vi "Initialize Page Number.vi"(8 "error in (no error)":errorcluster, 11 "Test Node Model in":refnum<class "Test Node Model.lvclass">) -> (0 "error out":errorcluster, 3 "Test Node Model out":refnum<class "Test Node Model.lvclass">)   [LabVIEW 2013, in "Test Node Model.lvlib" / "Test Node Model.lvclass"]
uses:
  Test Node Model.lvclass
  Test Node Model.lvclass/Test Node Model.ctl
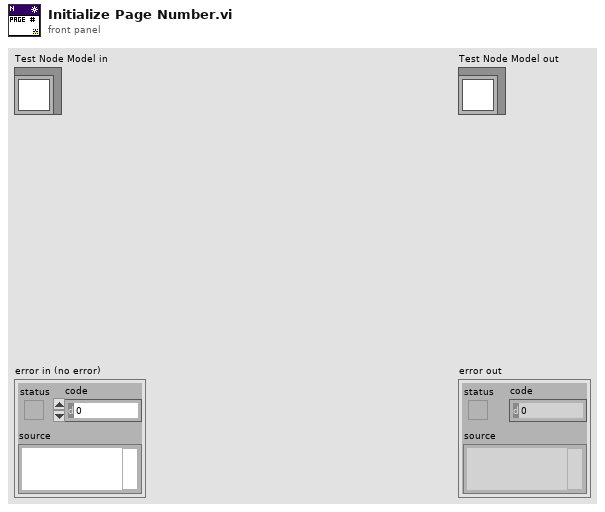
[diagram p1: front panel]
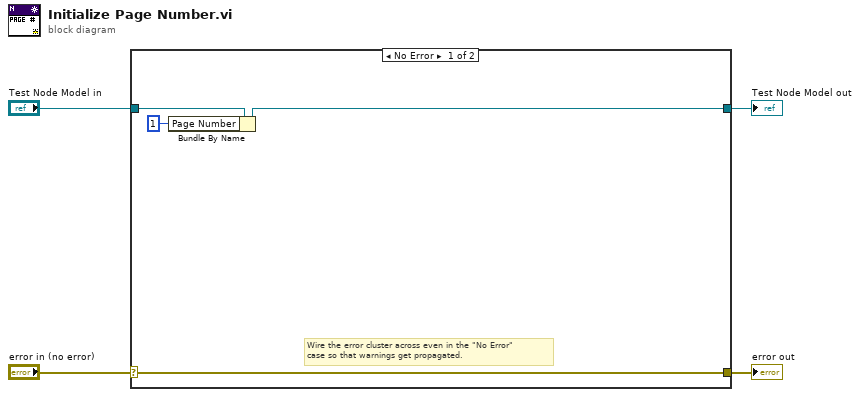
[diagram p0: block diagram]
diagram:
  n1 = case shown="No Error" "error in (no error)" {
    selector: "error in (no error)" -> [w7 w10]
    tunnel: [w7 w10] -> w3
    tunnel: [w6 w9] -> w1
    tunnel: "Test Node Model in" -> [w8 w9]
    frame No Error {
      # "Wire the error cluster across even in the \"No Error\"\ncase so that warnings get propagated."
      n2 = Bundle By Name(cluster=w8, "Page Number"=1) -> (w6:refnum<class "Test Node Model.lvclass">)
    }
    frame Error {
    }
  }
  "error out" <- w3
  "Test Node Model out" <- w1
